vi "GetConfigFile.vi"(4 "Tooling Pin Orientation":bool=TRUE, 5 "Stave Orientation":bool=TRUE, 6 "Build Configuration":T1={"Tape Type"=enum."Stereo (Sutcliffe Stave Core 8)", "Stave Coordinate System"=enum."Tooling Pins", "Module fiducial marker"=enum."Mark E (Slim/17)", "N Modules"=13}, 7 "base path":path=path "C:/Users/Aerotech/Documents/BNL_ThermomechanicalStave/ConfigFiles") -> (0 "ToolingPinOrientationString":string, 1 "StaveOrientationString":string, 2 "Stereo angle [mrad]":dbl, 3 "Stave Configuration File":path)   [LabVIEW 2016]
uses:
  Utils/Controls/BuildConfig.ctl
  Utils/Controls/All_Enums/Enum_TypeDef_TapeType.ctl
  Utils/Controls/All_Enums/Enum_TypeDef_StaveCalibMethod.ctl
  Utils/Controls/All_Enums/Enum_TypeDef_FidMarkers.ctl
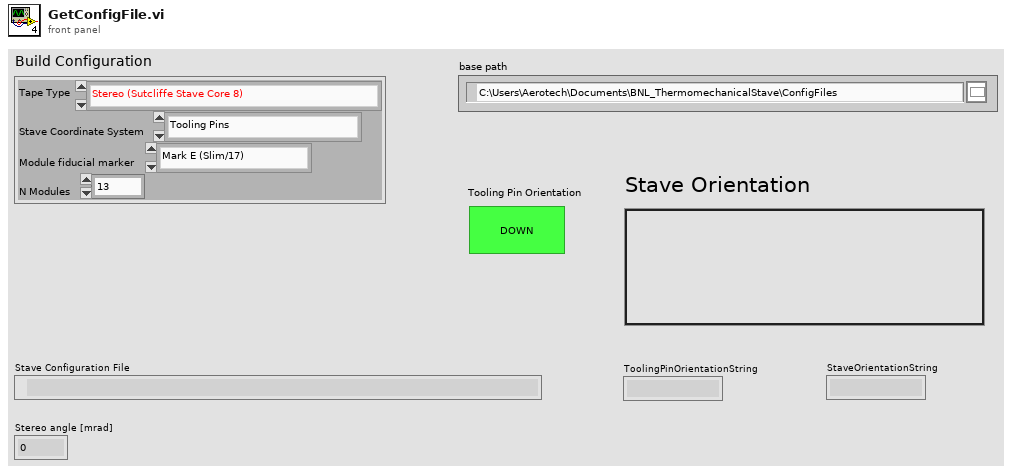
[diagram p1: front panel]
types:
  T1 = typedef "BuildConfig.ctl" = cluster{"Tape Type":T2, "Stave Coordinate System":T3, "Module fiducial marker":T4, "N Modules":i32}
  T2 = typedef "Enum_TypeDef_TapeType.ctl" = enum16{"Right stereo", "Left stereo", "Stereo (Sutcliffe NP49-01-100 01-Mar-16)", "Stereo (Sutcliffe 21-Jun-18- Electrical)", "Axial (Sutcliffe NP49-01-100 01-Mar-16)", "Stereo (Sutcliffe Stave Core 8)"}
  T3 = typedef "Enum_TypeDef_StaveCalibMethod.ctl" = enum16{"Tooling Pins", "Bus Tape"}
  T4 = typedef "Enum_TypeDef_FidMarkers.ctl" = enum16{"Mark B", "Mark C", "Bias Ring Corner", "Mark I (Slim/17)", "Mark E (Slim/17)", "Mark F (Slim/17)", "Mark G (Slim/17)", "Mark A (12)", "Kapton Spacers"}
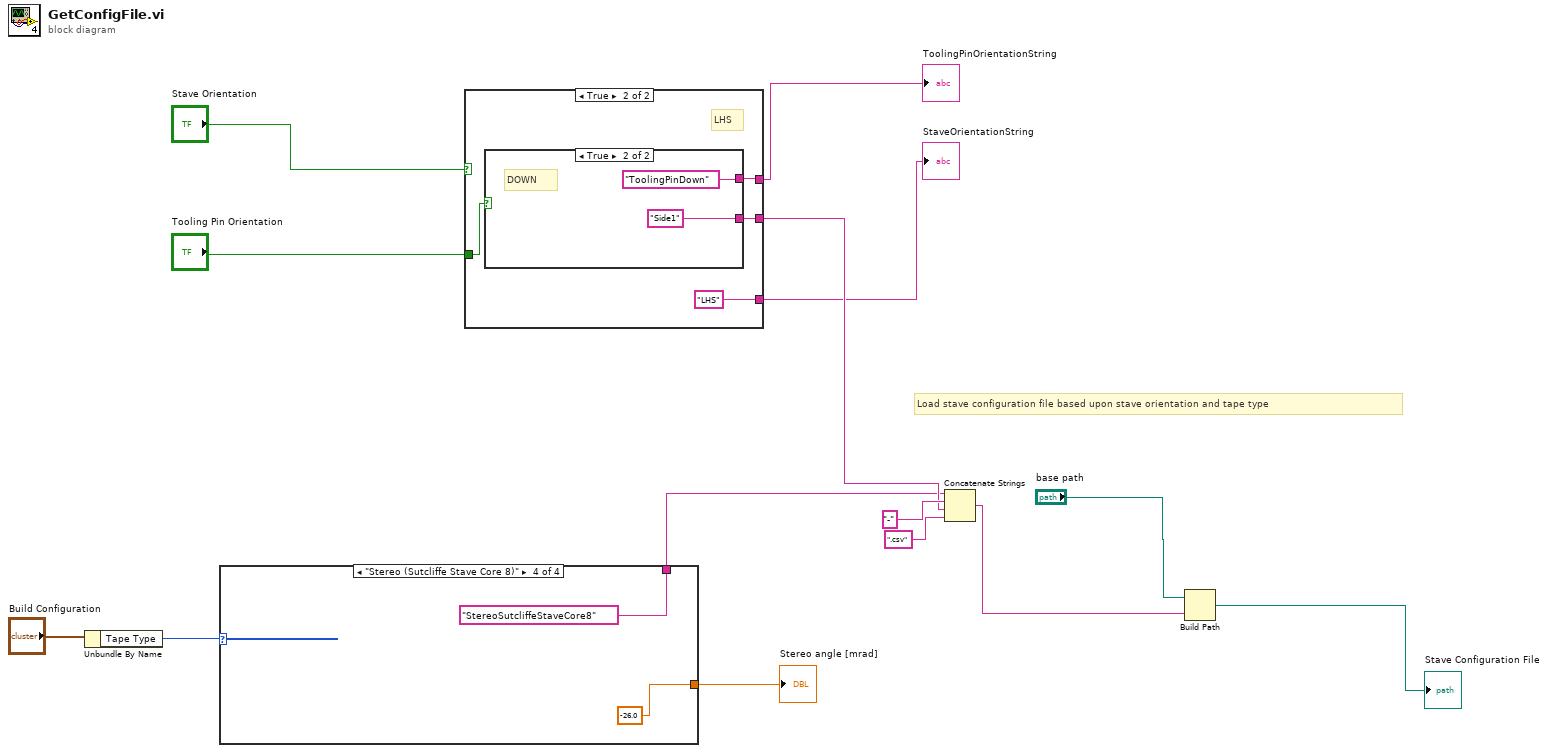
[diagram p0: block diagram]
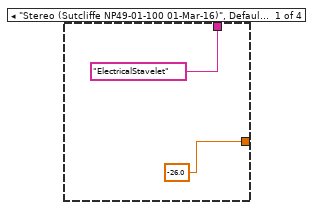
[diagram p2: hidden frame]
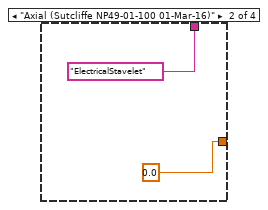
[diagram p3: hidden frame]
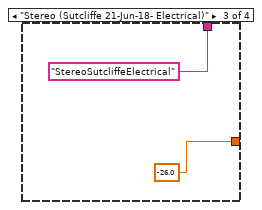
[diagram p4: hidden frame]
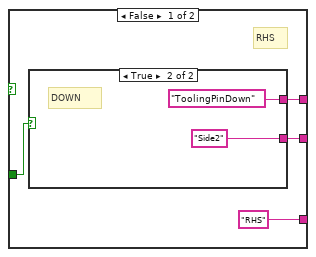
[diagram p5: hidden frame]
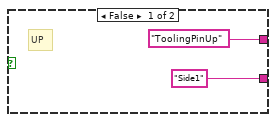
[diagram p6: hidden frame]
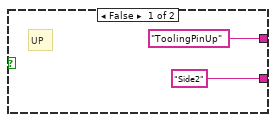
[diagram p7: hidden frame]
diagram:
  # "Load stave configuration file based upon stave orientation and tape type"
  n1 = Unbundle By Name("Build Configuration") -> ("Tape Type"=w5:T2)
  n2 = case shown="\"Stereo (Sutcliffe Stave Core 8)\"" w5 {
    tunnel: [-26.0 ("Stereo Angle [mrad]") 0.0 ("Stereo Angle [mrad]") -26.0 ("Stereo Angle [mrad]") -26.0 ("Stereo Angle [mrad]")] -> w4
    tunnel: ["ElectricalStavelet" "ElectricalStavelet" "StereoSutcliffeElectrical" "StereoSutcliffeStaveCore8"] -> w3
    frame "Stereo (Sutcliffe NP49-01-100 01-Mar-16)", Default {
    }
    frame "Axial (Sutcliffe NP49-01-100 01-Mar-16)" {
    }
    frame "Stereo (Sutcliffe 21-Jun-18- Electrical)" {
    }
    frame "Stereo (Sutcliffe Stave Core 8)" {
    }
  }
  "Stereo angle [mrad]" <- w4
  n3 = case shown="True" "Stave Orientation" {
    tunnel: "Tooling Pin Orientation" -> [w23 w31]
    tunnel: [w26 w34] -> w10
    tunnel: ["RHS" "LHS"] -> w1
    tunnel: [w24 w32] -> w2
    frame False {
      # "RHS"
      n4 = case shown="True" w23 {
        tunnel: ["Side1" "Side2"] -> w26
        tunnel: ["ToolingPinUp" "ToolingPinDown"] -> w24
        frame False {
          # "UP"
        }
        frame True {
          # "DOWN"
        }
      }
    }
    frame True {
      # "LHS"
      n5 = case shown="True" w31 {
        tunnel: ["Side2" "Side1"] -> w34
        tunnel: ["ToolingPinUp" "ToolingPinDown"] -> w32
        frame False {
          # "UP"
        }
        frame True {
          # "DOWN"
        }
      }
    }
  }
  "ToolingPinOrientationString" <- w2
  "StaveOrientationString" <- w1
  n6 = Concatenate Strings(w3, "-" ("string"), w10, ".csv" ("string")) -> (w7:string)
  n7 = Build Path(base path="base path", name or relative path=w7) -> (appended path=→"Stave Configuration File":path)
